vi "Generate Random String.vi"() -> (3 "Random String":string)   [LabVIEW 2023]
doc: "This subVI generates a random string of lowercase English characters whose length is between 1 and 10 characters."
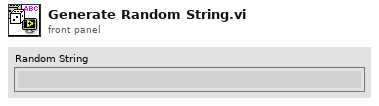
[diagram p1: front panel]
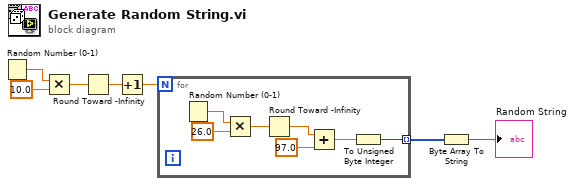
[diagram p0: block diagram]
diagram:
  n1 = Random Number (0-1)() -> (number: 0 to 1=w7:dbl)
  n2 = Multiply(x=w7, y=10.0) -> (x*y=w5:dbl)
  n3 = Round Toward -Infinity(1:w5) -> (0:w3:dbl)
  n4 = Increment(x=w3) -> (x+1=w4:dbl)
  n5 = for {
    N: w4 -> [_]
    tunnel: [w8] -> w2 mode=indexing
    n6 = Random Number (0-1)() -> (number: 0 to 1=w12:dbl)
    n7 = Multiply(x=w12, y=26.0) -> (x*y=w14:dbl)
    n8 = Round Toward -Infinity(1:w14) -> (0:w11:dbl)
    n9 = Add(x=w11, y=97.0) -> (x+y=w9:dbl)
    n10 = To Unsigned Byte Integer(number=w9) -> (unsigned 8bit integer=w8:u8)
  }
  n11 = Byte Array To String(unsigned byte array=w2) -> (string=→"Random String":string)
